vi "Receive.vi"   [LabVIEW 2025, in "ZeroMQ.lvlib" / "Socket.lvclass"]
uses:
  Socket.lvclass
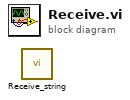
[diagram p0: block diagram]
diagram:
  n1 = call "Receive_string.vi"() -> ()  [unwired: 9 in, 3 out]
